vi "SQL_query.vi"(3 "error in (no error)":errorcluster, 4 "SQL query":string, 5 "联机模式":enum16{"单机", "追溯"}(ring)=enum."追溯") -> (0 "error out":errorcluster, 1 "data":string[][](array[string]))   [LabVIEW 2020]
uses:
  <vilib>/addons/database/Connection.llb/DB Tools Open Connec (String).vi
  <vilib>/addons/database/Connection.llb/Conn Execute.vi
  <vilib>/addons/database/Recordset.llb/Rec Fetch Recordset Data (R).vi
  <vilib>/addons/database/Recordset.llb/Rec Destroy - Connection.vi
  <vilib>/addons/database/NI_Database_API.lvlib
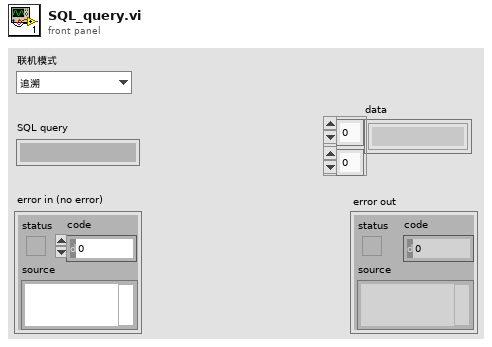
[diagram p1: front panel]
types:
  T1 = typedef "NI_Database_API.lvlib/Conn ObjectReference.ctl" = refnum<k1>
  T2 = typedef "NI_Database_API.lvlib/Rec ObjectReference.ctl" = refnum<k1>
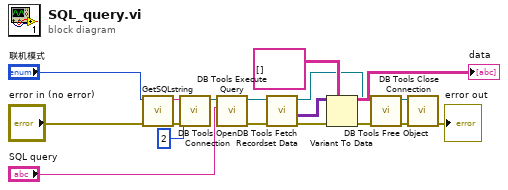
[diagram p0: block diagram]
diagram:
  n1 = call "GetSQLstring.vi"("错误输入"="error in (no error)", "联机模式"="联机模式") -> ("错误输出"=w8:errorcluster, "连接字符串"=w10:string)  [unwired: 8 in]
  n2 = call-poly <vilib>:"DB Tools Open Connection.vi"("error in (no error)"=w8, "connection timeout (15)"=2, "connection information"=w10) -> ("connection reference"=w12:T1)  [unwired: 5 in, 1 out]
  n3 = call-poly <vilib>:"DB Tools Execute Query.vi"("SQL query"="SQL query", "connection reference"=w12) -> ("error out"=w18:errorcluster, "recordset reference"=w17:T2)  [unwired: 6 in]
  n4 = call-poly <vilib>:"DB Tools Fetch Recordset Data.vi"("error in (no error)"=w18, "recordset reference"=w17) -> ("error out"=w16:errorcluster, "recordset data"=w15:variant[][], "recordset reference out"=w6:T2)  [unwired: 3 in]
  n5 = Variant To Data(error in=w16, type=string[][] [], Variant=w15) -> (data=→"data":string[][], error out=w5:errorcluster)
  n6 = call-poly <vilib>:"DB Tools Free Object.vi"("error in (no error)"=w5, "recordset reference"=w6) -> ("error out"=w3:errorcluster, "connection reference"=w4:T1)  [unwired: 8 in]
  n7 = call <vilib>:"DB Tools Close Connection.vi"("error in (no error)"=w3, "connection reference"=w4) -> ("error out"=→"error out":errorcluster)  [unwired: 5 in]
